vi "eFGV - Disabled Filter Index.vi"(6 "eFGV States":T1, 8 "Error In":errorcluster, 11 "Enabled Filter List":string[](array[string])) -> (0 "Error Out":errorcluster, 2 "Enabled Filter List Event":refnum<user-event>)   [LabVIEW 2020]
uses:
  Control/State - eFGV.ctl
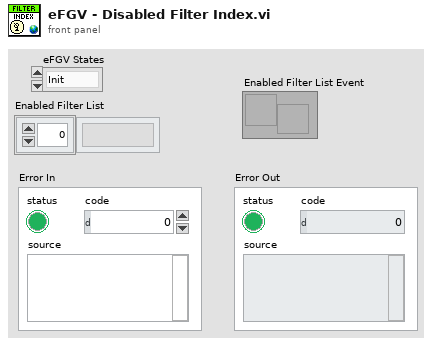
[diagram p1: front panel]
types:
  T1 = typedef "State - eFGV.ctl" = enum16{"Init", "Read", "Write", "Exit"}
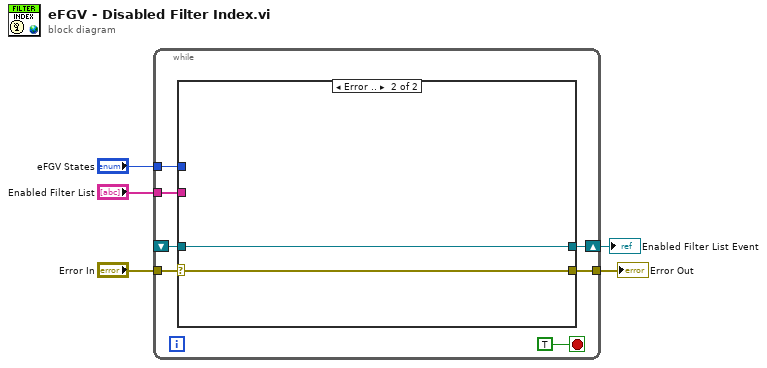
[diagram p0: block diagram]
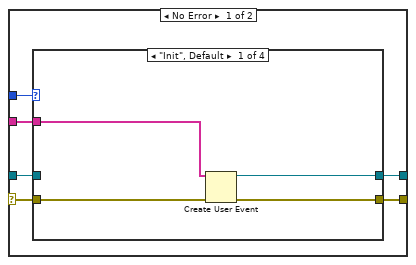
[diagram p2: hidden frame]
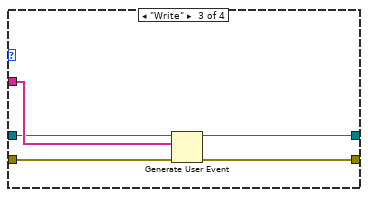
[diagram p4: hidden frame]
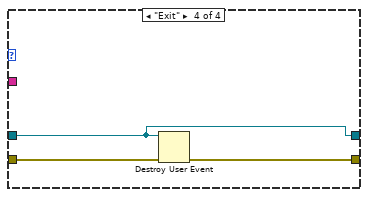
[diagram p5: hidden frame]
diagram:
  n1 = while {
    tunnel: "Error In" -> [w12]
    tunnel: "eFGV States" -> [w10]
    tunnel: [w9] -> w3
    tunnel: "Enabled Filter List" -> [w8]
    shift-right: [w7] -> w1
    shift-left: _ -> [w6]
    stop <- TRUE stop-if-true
    n2 = case shown="Error .." w12 {
      selector: w12 -> [w18 w34]
      tunnel: w10 -> [w17 _]
      tunnel: [w16 w34] -> w9
      tunnel: w8 -> [w15 _]
      tunnel: [w14 w33] -> w7
      tunnel: w6 -> [w13 w33]
      frame No Error {
        n3 = case shown="\"Init\", Default" w17 {
          tunnel: w18 -> [w22 w24 w29 w32]
          tunnel: [w21 w24 w28 w31] -> w16
          tunnel: w15 -> [w20 _ w27 _]
          tunnel: [w19 w23 w26 w30] -> w14
          tunnel: w13 -> [_ w23 w25 w30]
          frame "Init", Default {
            n4 = Create User Event(user event datatype=w20, error in=w22) -> (user event=w19:refnum<user-event>, error out=w21:errorcluster)
          }
          frame "Read" {
          }
          frame "Write" {
            n5 = Generate User Event(user event=w25, event data cluster=w27, error in=w29) -> (user event out=w26:refnum<user-event>, error out=w28:errorcluster)  [unwired: 1 in]
          }
          frame "Exit" {
            n6 = Destroy User Event(user event=w30, error in=w32) -> (error out=w31:errorcluster)
          }
        }
      }
      frame Error {
      }
    }
  }
  "Error Out" <- w3
  "Enabled Filter List Event" <- w1
